vi "XOR5.vi"(11 "inputs":T1={"Button 1"=TRUE, "Button 2"=TRUE, "Button 3"=TRUE, "Button 4"=TRUE, "Button 5"=FALSE}) -> (3 "XOR5":bool)   [LabVIEW 2014]
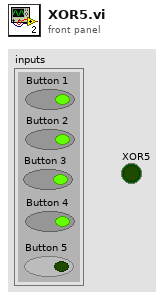
[diagram p1: front panel]
types:
  T1 = cluster{"Button 1":bool, "Button 2":bool, "Button 3":bool, "Button 4":bool, "Button 5":bool}
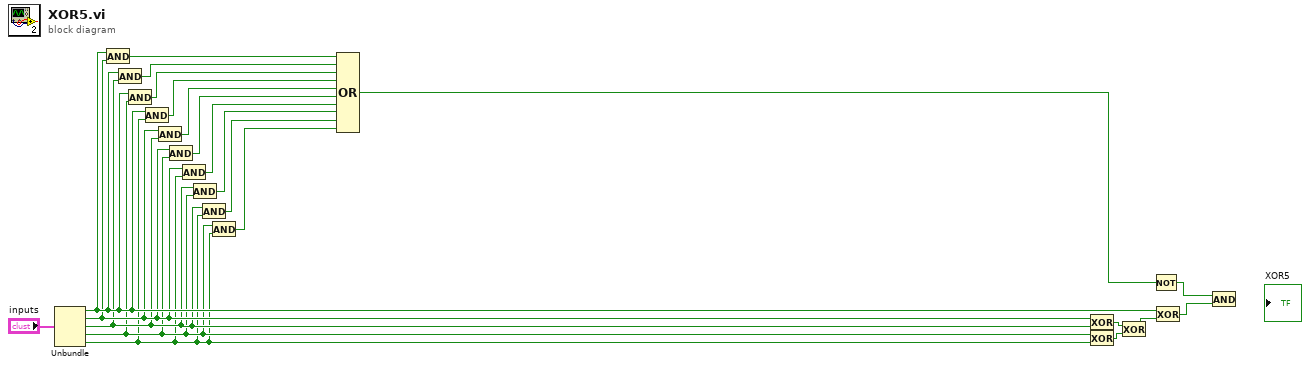
[diagram p0: block diagram]
diagram:
  n1 = Unbundle("inputs") -> ("Button 1"=w18:bool, "Button 2"=w17:bool, "Button 3"=w16:bool, "Button 4"=w15:bool, "Button 5"=w14:bool)
  n2 = And(x=w18, y=w17) -> (x .and. y?=w13:bool)
  n3 = And(x=w18, y=w16) -> (x .and. y?=w12:bool)
  n4 = And(x=w18, y=w15) -> (x .and. y?=w11:bool)
  n5 = And(x=w18, y=w14) -> (x .and. y?=w10:bool)
  n6 = And(x=w17, y=w16) -> (x .and. y?=w9:bool)
  n7 = And(x=w17, y=w15) -> (x .and. y?=w8:bool)
  n8 = And(x=w17, y=w14) -> (x .and. y?=w7:bool)
  n9 = And(x=w16, y=w15) -> (x .and. y?=w6:bool)
  n10 = And(x=w16, y=w14) -> (x .and. y?=w5:bool)
  n11 = And(x=w15, y=w14) -> (x .and. y?=w4:bool)
  n12 = Compound Arithmetic op=OR(w13, w12, w11, w10, w9, w8, w7, w6, w5, w4) -> (w3:bool)
  n13 = Exclusive Or(1:w16, 2:w17) -> (0:w22:bool)
  n14 = Exclusive Or(1:w14, 2:w15) -> (0:w21:bool)
  n15 = Exclusive Or(1:w21, 2:w22) -> (0:w20:bool)
  n16 = Not(x=w3) -> (.not. x?=w2:bool)
  n17 = Exclusive Or(1:w20, 2:w18) -> (0:w1:bool)
  n18 = And(x=w2, y=w1) -> ()  [unwired: 1 out]
